vi "Array-Subset by Endpoints.vi"() -> ()   [LabVIEW 2015]
panel:
  out "subarray":dbl[](array[numeric])
  in  "End Index":i32
  in  "Start Index":i32
  in  "Array":dbl[](array[numeric])
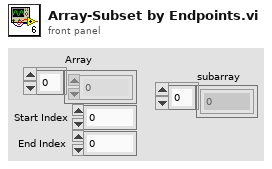
[diagram p1: front panel]
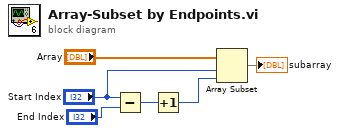
[diagram p0: block diagram]
diagram:
  n1 = Subtract(x="Start Index", y="End Index") -> (x-y=w5:i32)
  n2 = Increment(x=w5) -> (x+1=w2:i32)
  n3 = Array Subset(array="Array", index="Start Index", length=w2) -> (→"subarray":dbl[])
